vi "fibonacci_with_cache.vi"(9 "n":u16, 11 "cache in":map{u8, dbl}(c390)) -> (1 "F(n)":dbl, 3 "cache out":map{u8, dbl}(c390))   [LabVIEW 2021]
doc: "程序的说明请查看我的bl og： \nhttp://ruanqizhen.spaces.live.com/blog/cns!5852D4F797C53FB6!1832.entry"
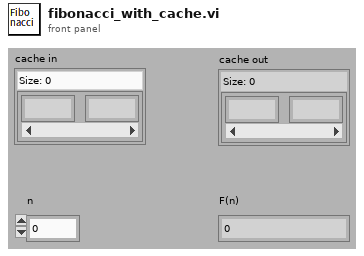
[diagram p1: front panel]
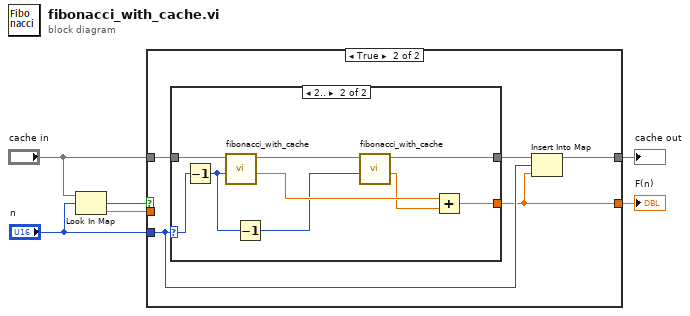
[diagram p0: block diagram]
diagram:
  n1 = Look In Map(map="cache in", key="n") -> (key not found?=w4:bool, value=w3:dbl)  [unwired: 1 in]
  n2 = case shown="True" w4 {
    tunnel: [w7 w10] -> w6
    tunnel: "n" -> [_ w11]
    tunnel: "cache in" -> [w8 w13]
    tunnel: [w8 w9] -> w5
    tunnel: w3 -> [w7 _]
    frame False {
    }
    frame True {
      n3 = case shown="2.." w11 {
        selector: w11 -> [w15 w24]
        tunnel: [w15 w23] -> w10
        tunnel: w13 -> [w14 w18]
        tunnel: [w14 w17] -> w12
        frame ..1, Default {
        }
        frame 2.. {
          n4 = Decrement(x=w24) -> (x-1=w16:u16)
          n5 = call "fibonacci_with_cache.vi"("n"=w16, "cache in"=w18) -> ("F(n)"=w22:dbl, "cache out"=w19:map{u8, dbl})  [unwired: 8 in]
          n6 = Decrement(x=w16) -> (x-1=w21:u16)
          n7 = call "fibonacci_with_cache.vi"("n"=w21, "cache in"=w19) -> ("F(n)"=w20:dbl, "cache out"=w17:map{u8, dbl})  [unwired: 8 in]
          n8 = Add(x=w22, y=w20) -> (x+y=w23:dbl)
        }
      }
      n9 = Insert Into Map(map in=w12, key=w11, value=w10) -> (map out=w9:map{u8, dbl})  [unwired: 2 out]
    }
  }
  "F(n)" <- w6
  "cache out" <- w5
